vi "Multi-Element ANN File Write.vi"(8 "File Error In":errorcluster, 10 "Array In":sgl[][](array[numeric]), 11 "Training refnum":refnum<file>) -> (0 "error out":errorcluster, 3 "refnum out":refnum<file>)   [LabVIEW 2020]
panel:
  out "error out 2":errorcluster
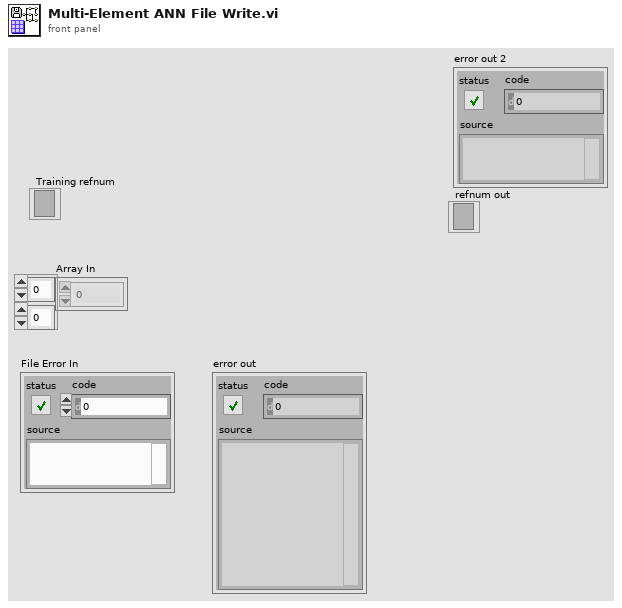
[diagram p1: front panel]
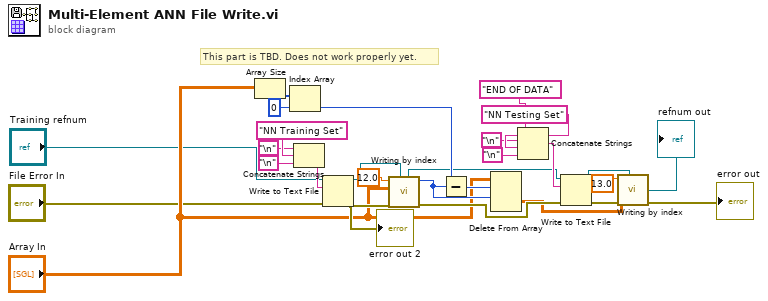
[diagram p0: block diagram]
diagram:
  # "This part is TBD. Does not work properly yet."
  n1 = Array Size(array="Array In") -> (size(s)=w14:i32[])
  n2 = Index Array(array=w14, index=0) -> (element=w16:i32)
  n3 = Concatenate Strings("\n", "NN Training Set" ("string"), "\n") -> (w10:string)
  n4 = Write to Text File(file (use dialog)="Training refnum", text=w10, error in="File Error In") -> (refnum out=w1:refnum<file>, error out=w17:errorcluster)  [unwired: 1 in, 1 out]
  "error out 2" <- w17
  n5 = call "Writing by index.vi"("refnum in"=w1, "error in"=w17, "Input array"="Array In", "While Equal to index"=sgl 12.0) -> ("error out"=w26:errorcluster, "Subarray Size"=w20:i32, "refnum out"=w3:refnum<file>)  [unwired: 3 in]
  n6 = Subtract(x=w16, y=w20) -> (x-y=w19:i32)
  n7 = Delete From Array(array="Array In", length=w19, index (row)=w20) -> (deleted portion=w6:sgl[][])  [unwired: 1 in, 1 out]
  n8 = Concatenate Strings("END OF DATA", "\n", "NN Testing Set" ("string"), "\n") -> (w27:string)
  n9 = Write to Text File(file (use dialog)=w3, text=w27, error in=w26) -> (refnum out=w25:refnum<file>, error out=→"error out":errorcluster)  [unwired: 1 in, 1 out]
  n10 = call "Writing by index.vi"("refnum in"=w25, "Input array"=w6, "While Equal to index"=sgl 13.0) -> ("refnum out"=→"refnum out":refnum<file>)  [unwired: 4 in, 2 out]
